vi "Write UI VI Reference.vi"(10 "UI VI Reference":refnum<vi>, 11 "Philips UI in":refnum<class "Flex UI.lvclass">) -> (3 "Philips UI out":refnum<class "Flex UI.lvclass">)   [LabVIEW 2014, in "Flex UI.lvclass"]
uses:
  Flex UI.lvclass
  Flex UI.lvclass/Flex UI.ctl
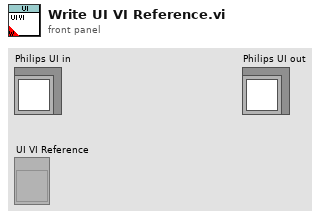
[diagram p1: front panel]
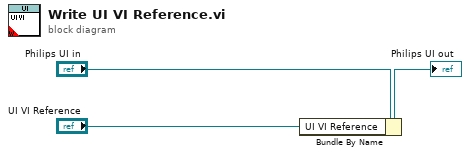
[diagram p0: block diagram]
diagram:
  n1 = Bundle By Name(cluster="Philips UI in", "UI VI Reference"="UI VI Reference") -> (→"Philips UI out":refnum<class "Flex UI.lvclass">)
